vi "Andor_Settings.vi"() -> ()   [LabVIEW 2018]
uses:
  <userlib>/atmcd32d.llb/HSSpeed_type typedef.ctl
panel:
  in  "OK Button":bool
  in  "Vertical clock voltage":i32(ring) items=["Normal", "+1", "+2", "+3", "+4"]
  in  "Shift speed":i32(ring) items=["0.564720", "1.016496", "1.920048", "[3.727152]"]
  in  "Readout rate":i32(ring) items=["35.00MHz", "27.00MHz", "13.00MHz"]
  in  "Pre-amplifier gain":i32(ring) items=["1.000000x", "1.900000x", "3.700000x"]
  in  "Binning":i32[](array[numeric])
  in  "ROI":i32[][](array[numeric])
  in  "EM Gain":u32 min=3
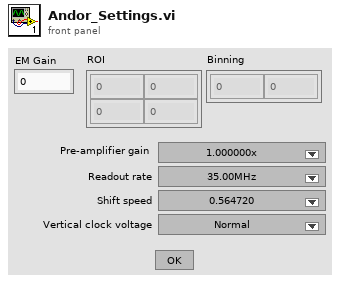
[diagram p1: front panel]
types:
  T1 = typedef "HSSpeed_type typedef.ctl" = enum16{"EM Amp", "Conventional Amp"}
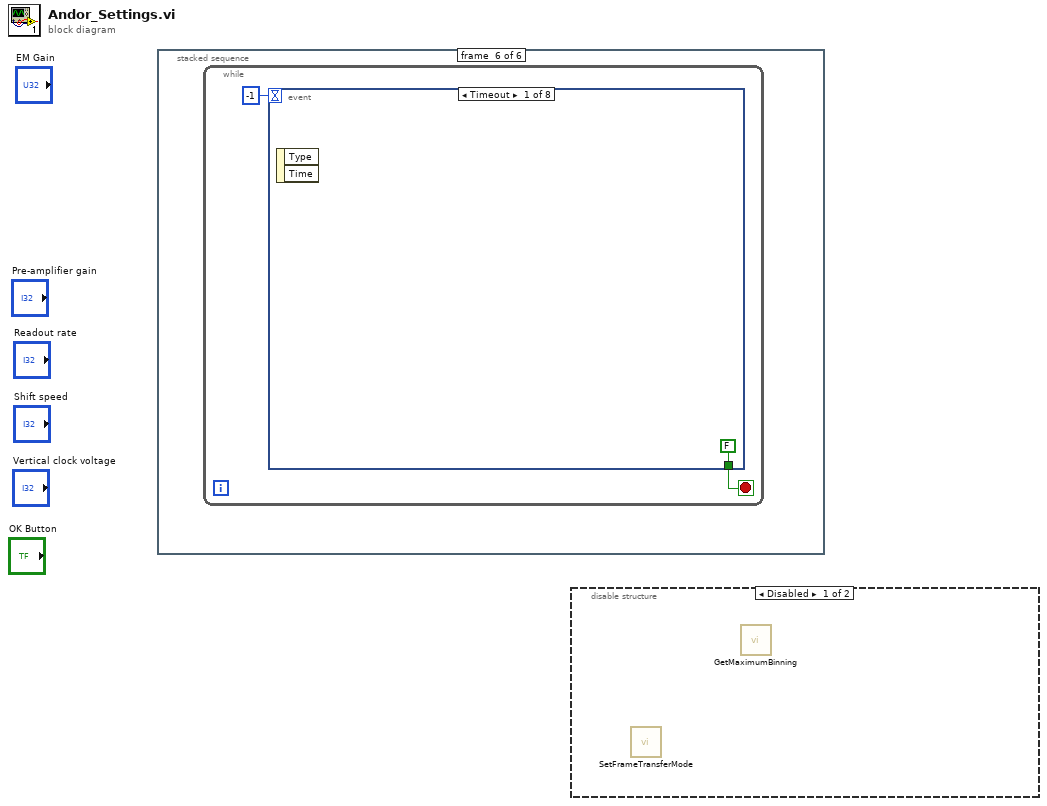
[diagram p0: block diagram]
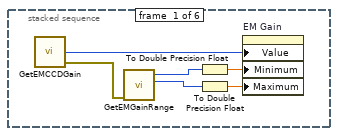
[diagram p3: hidden frame]
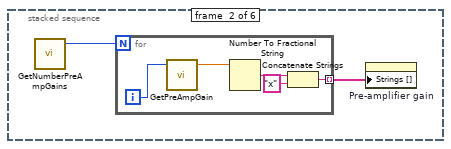
[diagram p4: hidden frame]
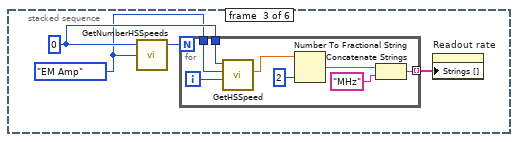
[diagram p5: hidden frame]
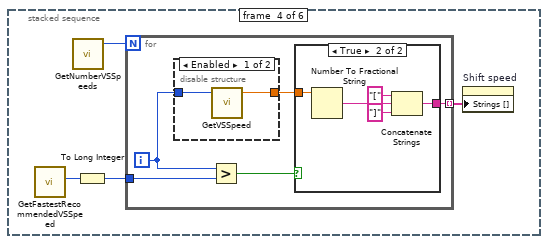
[diagram p6: hidden frame]
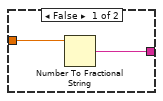
[diagram p7: hidden frame]
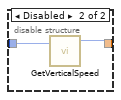
[diagram p8: hidden frame]
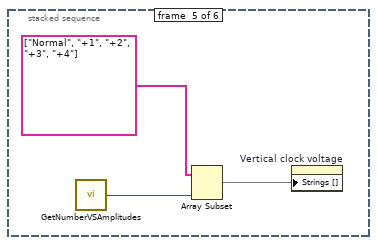
[diagram p9: hidden frame]
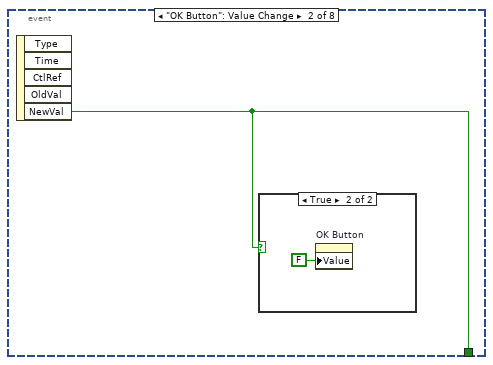
[diagram p10: hidden frame]
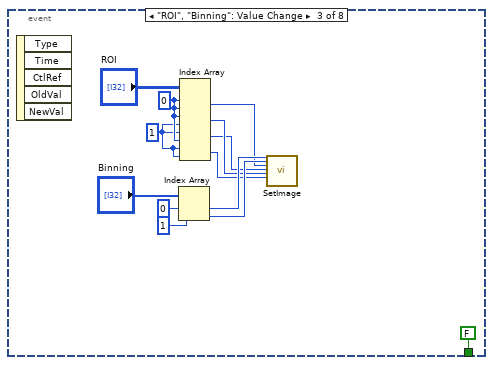
[diagram p12: hidden frame]
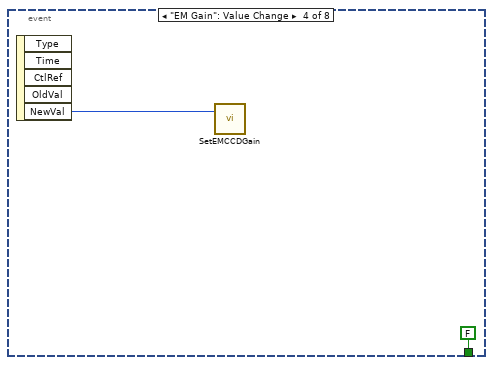
[diagram p13: hidden frame]
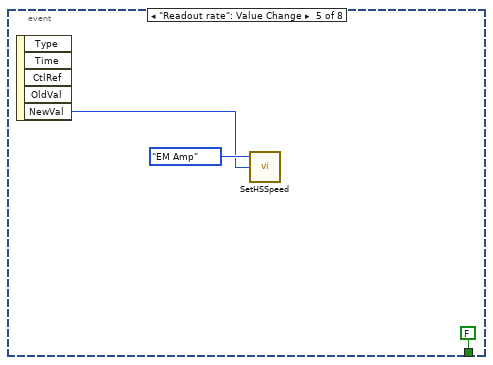
[diagram p14: hidden frame]
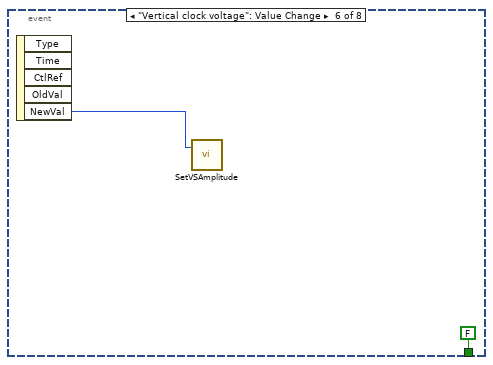
[diagram p15: hidden frame]
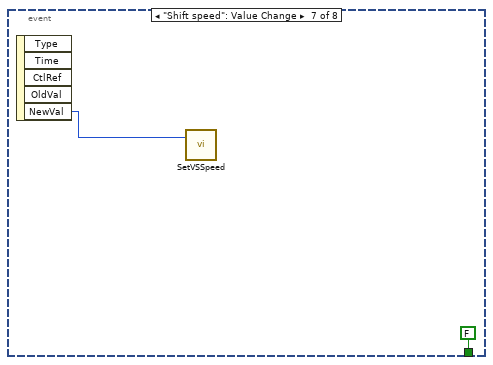
[diagram p16: hidden frame]
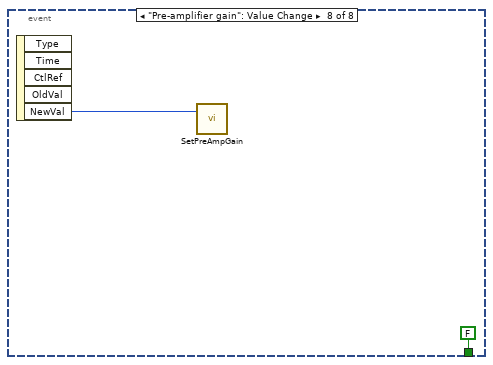
[diagram p17: hidden frame]
diagram:
  n1 = stacked-sequence {
    frame #0 {
      n2 = call <userlib>:"GetEMCCDGain.vi"() -> ("error out"=w3:errorcluster, "gain"=w6:u32)  [unwired: 3 in, 1 out]
      n3 = call <userlib>:"GetEMGainRange.vi"("error in (no error)"=w3) -> ("high"=w4:i32, "low"=w5:i32)  [unwired: 3 in, 2 out]
      n4 = To Double Precision Float(number=w5) -> (double precision float=w2:dbl)
      n5 = To Double Precision Float(number=w4) -> (double precision float=w1:dbl)
      n6 = property on="EM Gain" class="DigNum (strict)"("Value"=w6, "Minimum"=w2, "Maximum"=w1) -> ()  [unwired: 2 in, 2 out]
    }
    frame #1 {
      n7 = call <userlib>:"GetNumberPreAmpGains.vi"() -> ("number"=w7:i32)  [unwired: 3 in, 2 out]
      n8 = for {
        N: w7 -> [_]
        tunnel: [w11] -> w8 mode=indexing
        i -> [w10]
        n9 = call <userlib>:"GetPreAmpGain.vi"("index"=w10) -> ("gain"=w9:sgl)  [unwired: 2 in, 2 out]
        n10 = Number To Fractional String(number=w9) -> (F-format string=w13:string)  [unwired: 3 in]
        n11 = Concatenate Strings(w13, "x" ("string")) -> (w11:string)
      }
      n12 = property on="Pre-amplifier gain" class="Ring (strict)"("Strings []"=w8) -> ()  [unwired: 2 in, 2 out]
    }
    frame #2 {
      w14 = HSSpeed_type_typedef."EM Amp" ("type")
      w15 = 0 ("channel")
      n13 = call <userlib>:"GetNumberHSSpeeds.vi"("type"=w14, "channel"=w15) -> ("number"=w16:i32)  [unwired: 1 in, 2 out]
      n14 = for {
        N: w16 -> [_]
        tunnel: [w23] -> w17 mode=indexing
        tunnel: w15 -> [w20]
        tunnel: w14 -> [w19]
        i -> [w21]
        n15 = call <userlib>:"GetHSSpeed.vi"("index"=w21, "type"=w19, "channel"=w20) -> ("speed"=w22:sgl)  [unwired: 2 in, 2 out]
        n16 = Number To Fractional String(number=w22, precision (6)=i16 2) -> (F-format string=w25:string)  [unwired: 2 in]
        n17 = Concatenate Strings(w25, "MHz" ("string")) -> (w23:string)
      }
      n18 = property on="Readout rate" class="Ring (strict)"("Strings []"=w17) -> ()  [unwired: 2 in, 2 out]
    }
    frame #3 {
      n19 = call <userlib>:"GetFastestRecommendedVSSpeed.vi"() -> ("index"=w27:u32)  [unwired: 4 in, 3 out]
      n20 = call <userlib>:"GetNumberVSSpeeds.vi"() -> ("number"=w28:i32)  [unwired: 3 in, 2 out]
      n21 = To Long Integer(number=w27) -> (32bit integer=w26:i32)
      n22 = for {
        N: w28 -> [_]
        tunnel: [w33] -> w29 mode=indexing
        tunnel: w26 -> [w31]
        i -> [w32]
        n23 = disable-structure shown="Enabled" {
          disable-tunnel: [w42 w44] -> w34
          disable-tunnel: w32 -> [w43 w45]
          frame Enabled {
            n24 = call <userlib>:"GetVSSpeed.vi"("index"=w43) -> ("speed"=w42:sgl)  [unwired: 2 in, 2 out]
          }
          frame Disabled {
            n25 = call <userlib>:"GetVerticalSpeed.vi"("index"=w45) -> ("speed"=w44:i32)  [unwired: 1 in, 2 out]
          }
        }
        n26 = Greater?(x=w32, y=w31) -> (0:w30:bool)
        n27 = case shown="True" w30 {
          tunnel: w34 -> [w36 w41]
          tunnel: [w35 w39] -> w33
          frame False {
            n28 = Number To Fractional String(number=w36) -> (F-format string=w35:string)  [unwired: 3 in]
          }
          frame True {
            n29 = Number To Fractional String(number=w41) -> (F-format string=w40:string)  [unwired: 3 in]
            n30 = Concatenate Strings("[" ("string"), w40, "]" ("string")) -> (w39:string)
          }
        }
      }
      n31 = property on="Shift speed" class="Ring (strict)"("Strings []"=w29) -> ()  [unwired: 2 in, 2 out]
    }
    frame #4 {
      n32 = call <userlib>:"GetNumberVSAmplitudes.vi"() -> ("number"=w46:i32)  [unwired: 3 in, 2 out]
      n33 = Array Subset(array=string[] ["Normal", "+1", "+2", "+3", "+4"], length=w46) -> (w47:string[])  [unwired: 1 in]
      n34 = property on="Vertical clock voltage" class="Ring (strict)"("Strings []"=w47) -> ()  [unwired: 2 in, 2 out]
    }
    frame #5 {
      n35 = while {
        stop <- w49 stop-if-true
        n36 = event shown="[0] Timeout" {
          selector: _ -> [_ _ _ _ _ _ _ _]
          dyn-events: _ -> [_ _ _ _ _ _ _ _]
          timeout: -1 -> [_ _ _ _ _ _ _ _]
          tunnel: [FALSE ("NewVal") w52 FALSE ("NewVal") FALSE ("NewVal") FALSE ("NewVal") FALSE ("NewVal") FALSE ("NewVal") FALSE ("NewVal")] -> w49
          event Timeout {
            n37 = event-data() -> ()  [unwired: 1 in, 2 out]
          }
          event "OK Button": Value Change {
            n38 = event-data() -> ("NewVal"=w52:bool)  [unwired: 1 in, 4 out]
            n39 = case shown="True" w52 {
              frame False {
              }
              frame True {
                n40 = property on="OK Button" class="Bool (strict)"("Value"=FALSE ("OK Button")) -> ()  [unwired: 2 in, 2 out]
              }
            }
          }
          event "ROI", "Binning": Value Change {
            w58 = 1 ("index (row)")
            w59 = 0 ("index (row)")
            n41 = event-data() -> ()  [unwired: 1 in, 5 out]
            n42 = Index Array(array="Binning", index #1=0 ("index"), index #2=1 ("index")) -> (element #1=w64:i32, element #2=w61:i32)
            n43 = Index Array(array="ROI", index (row) #1=w59, index (col) #1=w59, index (row) #2=w59, index (col) #2=w58, index (row) #3=w58, index (col) #3=w59, index (row) #4=w58, index (col) #4=w58) -> (element #1=w57:i32, element #2=w56:i32, element #3=w54:i32, element #4=w55:i32)
            n44 = call <userlib>:"SetImage.vi"("hbin"=w64, "vbin"=w61, "hstart"=w57, "hend"=w54, "vstart"=w56, "vend"=w55) -> ()  [unwired: 20 in, 2 out]
          }
          event "EM Gain": Value Change {
            n45 = event-data() -> ("NewVal"=w67:u32)  [unwired: 1 in, 4 out]
            n46 = call <userlib>:"SetEMCCDGain.vi"("gain"=w67) -> ()  [unwired: 1 in, 2 out]
          }
          event "Readout rate": Value Change {
            n47 = event-data() -> ("NewVal"=w70:i32)  [unwired: 1 in, 4 out]
            n48 = call <userlib>:"SetHSSpeed.vi"("index"=w70, "type"=HSSpeed_type_typedef."EM Amp") -> ()  [unwired: 2 in, 2 out]
          }
          event "Vertical clock voltage": Value Change {
            n49 = event-data() -> ("NewVal"=w73:i32)  [unwired: 1 in, 4 out]
            n50 = call <userlib>:"SetVSAmplitude.vi"("amplitude"=w73) -> ()  [unwired: 1 in, 2 out]
          }
          event "Shift speed": Value Change {
            n51 = event-data() -> ("NewVal"=w75:i32)  [unwired: 1 in, 4 out]
            n52 = call <userlib>:"SetVSSpeed.vi"("index"=w75) -> ()  [unwired: 1 in, 2 out]
          }
          event "Pre-amplifier gain": Value Change {
            n53 = event-data() -> ("NewVal"=w77:i32)  [unwired: 1 in, 4 out]
            n54 = call <userlib>:"SetPreAmpGain.vi"("index"=w77) -> ()  [unwired: 1 in, 2 out]
          }
        }
      }
    }
  }
  n55 = disable-structure shown="Disabled" {
    frame Disabled {
      n56 = call <userlib>:"SetFrameTransferMode.vi"() -> ()  [unwired: 2 in, 2 out]
      n57 = call <userlib>:"GetMaximumBinning.vi"() -> ()  [unwired: 3 in, 3 out]
    }
    frame Enabled {
    }
  }
